vi "GetSeededSwerveAzimuth.vi"(8 "Calibration Occured":bool, 9 "Falcon Brownout Occured":bool, 10 "Relative Position (Raw Sensor Units)":i32, 11 "Absolute Position Seed (deg) [-180,+180]":dbl) -> (2 "Azimuth Position (deg) [-180,+180]":dbl)   [LabVIEW 2019]
uses:
  f4340844-ff0c-4785-83bc-3e3f8e66c499.vi
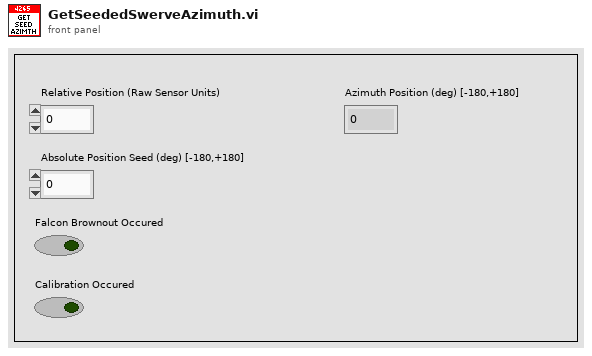
[diagram p1: front panel]
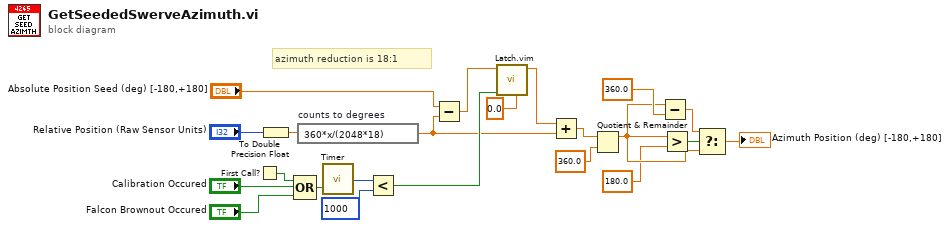
[diagram p0: block diagram]
diagram:
  # "azimuth reduction is 18:1"
  n1 = First Call?() -> (First Call?: T/F=w16:bool)
  n2 = To Double Precision Float(number="Relative Position (Raw Sensor Units)") -> (double precision float=w7:dbl)
  n3 = Compound Arithmetic op=OR(w16, "Calibration Occured", "Falcon Brownout Occured") -> (w17:bool)
  n4 = expression code="360*x/(2048*18)" "counts to degrees"(w7) -> (w13:dbl)
  n5 = call "Timer.vi"("Reset Timer"=w17) -> ("Time (ms)"=w14:u32)
  n6 = Less?(x=w14, y=u32 1000) -> (x < y?=w18:bool)
  n7 = Subtract(x="Absolute Position Seed (deg) [-180,+180]", y=w13) -> (x-y=w9:dbl)
  n8 = call "Latch.vim"("Default Value"=0.0, "Latch Signal"=w18, "Latch Value"=w9) -> ("Latched"=w11:dbl)  [unwired: 8 in]
  n9 = Add(x=w11, y=w13) -> (x+y=w10:dbl)
  n10 = Quotient & Remainder(x=w10, y=360.0) -> (x-y*floor(x/y)=w4:dbl)  [unwired: 1 out]
  n11 = Subtract(x=w4, y=360.0) -> (x-y=w5:dbl)
  n12 = Greater?(x=w4, y=180.0) -> (0:w3:bool)
  n13 = Select(t=w5, s=w3, f=w4) -> (s? t:f=→"Azimuth Position (deg) [-180,+180]":dbl)
